vi "Get All Paths in Variant.vi"(8 "error in (no error)":errorcluster, 11 "Variant":variant) -> (0 "error out":errorcluster, 3 "Paths out":string[](array[string]))   [LabVIEW 2017, in "Advanced Variant Tools.lvlib"]
uses:
  Advanced Variant Tools.lvlib
  <vilib>/Utility/Data Type/NI_Data Type.lvlib
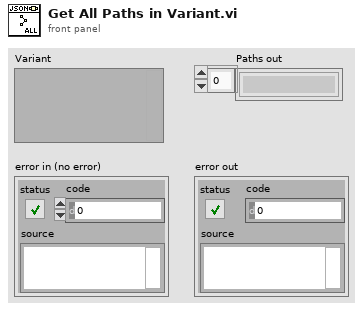
[diagram p1: front panel]
types:
  T1 = typedef "NI_Data Type.lvlib/Data Type.ctl" = enum8{"Invalid Type", "Void", "I8", "I16", "I32", "I64", "U8", "U16", "U32", "U64", "Single Float", "Double Float", "Extended Float", "Single Complex", "Double Complex", "Extended Complex", "Enum U8", "Enum U16", "Enum U32", "Enum U64", "Single Float With Unit", "Double Float With Unit", "Extended Float With Unit", "Single Complex with Unit", "Double Complex with Unit", "Extended Complex with Unit", "Boolean", "String", "Path", "Picture", "Tag", "Array", "Cluster", "Variant", "LV Variant", "Waveform", "Timestamp", "Digital Waveform", "Digital Data", "ExpressData", "Refnum", "External Data", "VI", "Poly VI", "LabVIEW Class Instance", "Fixed Point"}
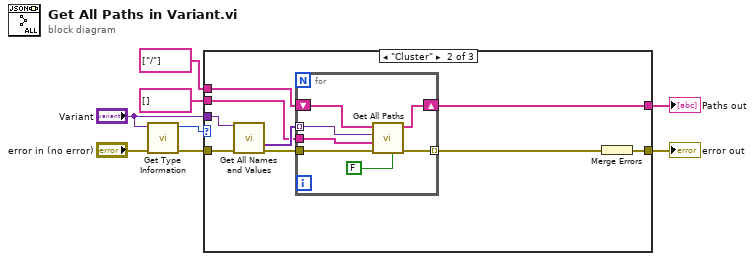
[diagram p0: block diagram]
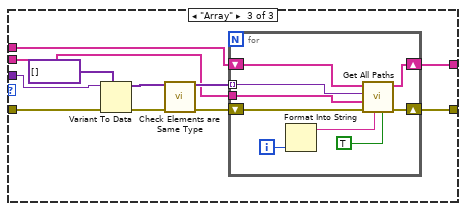
[diagram p3: hidden frame]
diagram:
  n1 = call <vilib>:"Get Type Information.vi"("error in (no error)"="error in (no error)", "Variant"="Variant") -> ("error out"=w1:errorcluster, "Type"=w3:T1)  [unwired: 5 in, 3 out]
  n2 = case shown="\"Cluster\"" w3 {
    tunnel: w1 -> [w10 w12 w33]
    tunnel: [w10 w16 w37] -> w5
    tunnel: "Variant" -> [_ w19 w35]
    tunnel: string[] [] ("Array 3") -> [_ w15 w29]
    tunnel: string[] ["/"] ("Paths in") -> [w9 w14 w28]
    tunnel: [w9 w13 w27] -> w8
    frame Default {
    }
    frame "Cluster" {
      n3 = call "Get All Names and Values.vi"("Variant (Cluster) In"=w19, "error in"=w12) -> ("Values"=w18:variant[], "error out"=w11:errorcluster)  [unwired: 9 in, 3 out]
      n4 = for {
        tunnel: w18 -> [w26] mode=indexing
        tunnel: [w25] -> w17 mode=indexing
        shift-right: [w20] -> w13
        shift-left: w14 -> [w21]
        tunnel: w11 -> [w23]
        tunnel: w15 -> [w22]
        n5 = call "Get All Paths.vi"("is array element?"=FALSE ("first call?"), "error in (no error)"=w23, "parents"=w22, "Variant"=w26, "Paths"=w21) -> ("error out"=w25:errorcluster, "Paths out"=w20:string[])  [unwired: 5 in]
      }
      n6 = Merge Errors(w17) -> (w16:errorcluster)
    }
    frame "Array" {
      n7 = Variant To Data(error in=w33, type=variant[] [], Variant=w35) -> (data=w34:variant[], error out=w32:errorcluster)
      n8 = call "Check Elements are Same Type.vi"("array in"=w34, "error in (no error)"=w32) -> ("array out"=w31:variant[], "error out"=w30:errorcluster)  [unwired: 12 in]
      n9 = for {
        tunnel: w31 -> [w43] mode=indexing
        shift-right: [w46] -> w37
        shift-left: w30 -> [w45]
        shift-right: [w39] -> w27
        shift-left: w28 -> [w38]
        tunnel: w29 -> [w40]
        i -> [w42]
        n10 = Format Into String(w42) -> (resulting string=w41:string)  [unwired: 3 in, 1 out]
        n11 = call "Get All Paths.vi"("is array element?"=TRUE ("first call?"), "index string"=w41, "error in (no error)"=w45, "parents"=w40, "Variant"=w43, "Paths"=w38) -> ("error out"=w46:errorcluster, "Paths out"=w39:string[])  [unwired: 4 in]
      }
    }
  }
  "Paths out" <- w8
  "error out" <- w5
